vi "validacion A-D.vi"(8 "error in (no error)":errorcluster, 11 "ID":i32) -> (0 "error out":errorcluster, 2 "rate":dbl, 3 "Tiempo":i32, 4 "Digital Signal":T1={"DAQ Board Name"="DAQ_Simu1", "Port Digitales"=[], "rate"=1000.0, "Tiempo"=100}, 6 "Type Signal":T2={"DAQ Board Name"="DAQ_Simu1", "Analogicos Canales"=["DAQ_Simu1/ai1", "DAQ_Simu1/ai2"], "rate"=1000.0, "number of samples "=1000, "Tiempo"=100})   [LabVIEW 2020, in "Settings.lvlib"]
uses:
  Settings.lvlib
  typeSignal--cluster.ctl
  Digital typeSignal--cluster.ctl
  <vilib>/drjdpowell/SQLite Library/SQL Connection/Open (path).vi
  <vilib>/drjdpowell/SQLite Library/SQL Connection/Open (string).vi
  <vilib>/AdvancedString/Path To Command Line String.vi
  <vilib>/drjdpowell/SQLite Library/SQL Connection/Execute SQL (1D UTF-8).vi
  <vilib>/drjdpowell/SQLite Library/SQL Connection/Connection.lvclass
  <vilib>/drjdpowell/SQLite Library/SQLite.lvlib
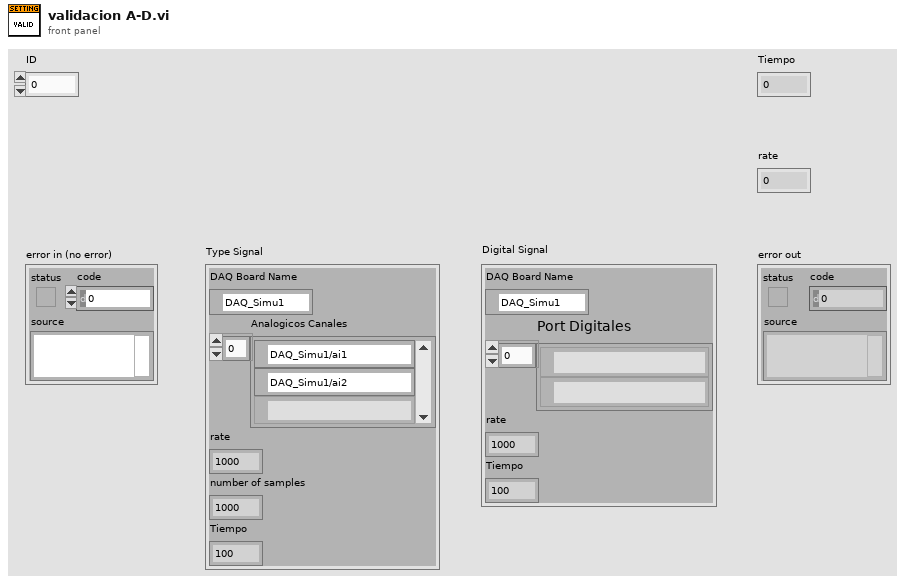
[diagram p1: front panel]
types:
  T1 = typedef "Digital typeSignal--cluster.ctl" = cluster{"DAQ Board Name":tag, "Port Digitales":tag[], "rate":dbl, "Tiempo":i32}
  T2 = typedef "typeSignal--cluster.ctl" = cluster{"DAQ Board Name":tag, "Analogicos Canales":tag[], "rate":dbl, "number of samples ":i32, "Tiempo":i32}
  T3 = cluster{"Result Set (UTF-8)[0]":string, "Result Set (UTF-8)[1]":string, "Result Set (UTF-8)[2]":string, "Result Set (UTF-8)[3]":string, "Result Set (UTF-8)[4]":string, "Result Set (UTF-8)[5]":string, "Result Set (UTF-8)[6]":string, "Result Set (UTF-8)[7]":string, "Result Set (UTF-8)[8]":string}
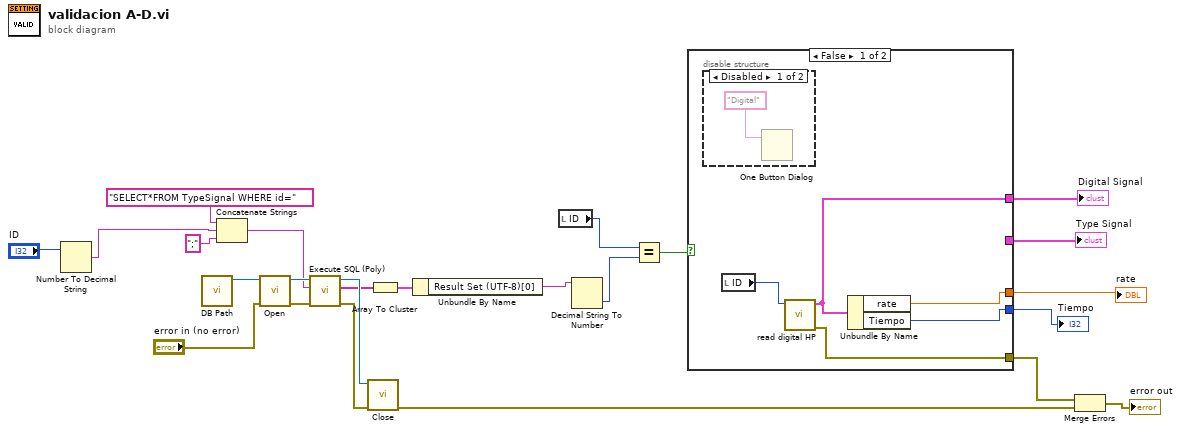
[diagram p0: block diagram]
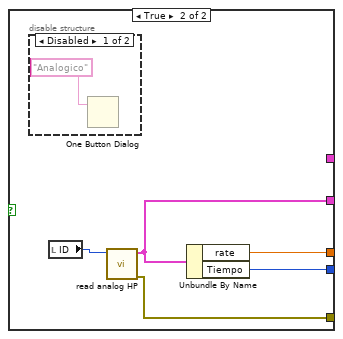
[diagram p3: hidden frame]
diagram:
  n1 = Number To Decimal String(number="ID") -> (decimal integer string=w11:string)  [unwired: 1 in]
  n2 = call "DB Path.vi"() -> ("DB path"=w16:path)  [unwired: 11 in]
  n3 = Concatenate Strings("SELECT*FROM TypeSignal WHERE id=" ("SQL"), w11, ";" ("string")) -> (w13:string)
  n4 = call-poly <vilib>:"Open.vi"("error in (no error)"="error in (no error)", "db file"=w16) -> ("error out"=w24:errorcluster, "SQLite Connection"=w23:refnum<class "Connection.lvclass">)  [unwired: 8 in]
  n5 = call-poly <vilib>:"Execute SQL (Poly).vi"("error in (no error)"=w24, "SQL"=w13, "SQLite Connection in"=w23) -> ("error out"=w21:errorcluster, "Result Set (UTF-8)"=w17:string[], "SQLite Connection"=w22:refnum<class "Connection.lvclass">)  [unwired: 5 in, 1 out]
  n6 = call-dynamic "Close.vi"("error in (no error)"=w21, "SQLite Connection in"=w22) -> ("error out"=w20:errorcluster)  [unwired: 9 in]
  n7 = Array To Cluster(array=w17) -> (cluster=w18:T3)
  n8 = Unbundle By Name(w18) -> ("Result Set (UTF-8)[0]"=w9:string)
  n9 = local read "ID"() -> (w10:i32)
  n10 = Decimal String To Number(string=w9) -> (number=w8:i32)  [unwired: 2 in, 1 out]
  n11 = Equal?(x=w10, y=w8) -> (x = y?=w7:bool)
  n12 = case shown="False" w7 {
    tunnel: [w25 w34] -> w5
    tunnel: [w27 w33] -> w4
    tunnel: [w26 w32] -> w3
    tunnel: [_ w31] -> w2
    tunnel: [w28 _] -> w1
    frame False {
      n13 = disable-structure shown="Disabled" {
        frame Disabled {
          n14 = One Button Dialog(message="Digital") -> ()  [unwired: 1 in, 1 out]
        }
        frame Enabled {
        }
      }
      n15 = local read "ID"() -> (w29:i32)
      n16 = call "read digital HP.vi"("ID"=w29) -> ("error out"=w25:errorcluster, "Digital Signal"=w28:T1)  [unwired: 9 in]
      n17 = Unbundle By Name(w28) -> ("rate"=w27:dbl, "Tiempo"=w26:i32)
    }
    frame True {
      n18 = disable-structure shown="Disabled" {
        frame Disabled {
          n19 = One Button Dialog(message="Analogico") -> ()  [unwired: 1 in, 1 out]
        }
        frame Enabled {
        }
      }
      n20 = local read "ID"() -> (w35:i32)
      n21 = call "read analog HP.vi"("ID"=w35) -> ("error out"=w34:errorcluster, "Type Signal"=w31:T2)  [unwired: 9 in]
      n22 = Unbundle By Name(w31) -> ("rate"=w33:dbl, "Tiempo"=w32:i32)
    }
  }
  "Tiempo" <- w3
  "rate" <- w4
  "Type Signal" <- w2
  "Digital Signal" <- w1
  n23 = Merge Errors(w5, w20) -> (→"error out":errorcluster)
